vi "DistortImageARGB.vi"(7 "Use Fixed Point Remapping (Default: False)":bool, 8 "error in (no error)":errorcluster, 9 "ARGB Image Destination":refnum<data-value>, 10 "ARGB Image Source":refnum<data-value>, 11 "ImageDistorter":refnum<class "ImageDistorter.lvclass">) -> (0 "error out":errorcluster, 2 "ARGB Image Destination (duplicate)":refnum<data-value>, 3 "ImageDistorter (Duplicate)":refnum<class "ImageDistorter.lvclass">)   [LabVIEW 2020, in "g_ar_toolkit.image.lvlib" / "ImageDistorter.lvclass"]
uses:
  ImageDistorter.lvclass
  ImageDistorter.lvclass/ImageDistorter.ctl
  ccc224f2-fea8-4097-85c8-c2b3fe04188f.vi
  g_ar_toolkit.common/Module Path.vi
  <vilib>/Utility/error.llb/Error Cluster From Error Code.vi
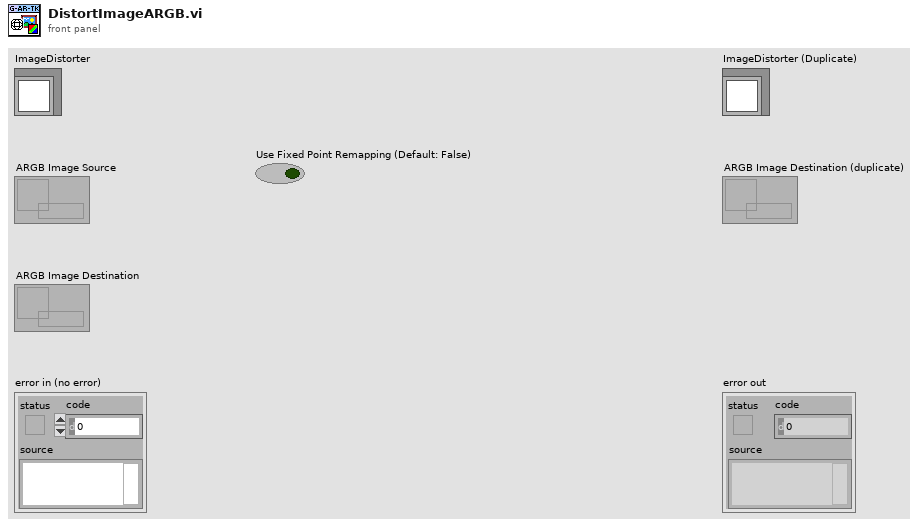
[diagram p1: front panel]
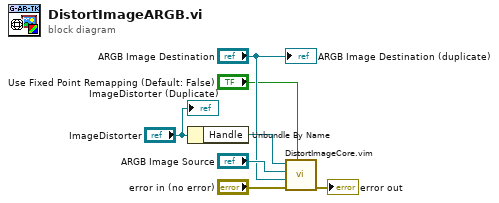
[diagram p0: block diagram]
diagram:
  n1 = Unbundle By Name("ImageDistorter") -> ("Handle"=w6:refnum<data-value>)
  n2 = call "DistortImageCore.vim"("Use Fixed Point remapping"="Use Fixed Point Remapping (Default: False)", "error in (no error)"="error in (no error)", "Destination Image"="ARGB Image Destination", "Source Image"="ARGB Image Source", "Handle"=w6) -> ("error out"=→"error out":errorcluster)  [unwired: 6 in]
  "ImageDistorter (Duplicate)" <- "ImageDistorter"
  "ARGB Image Destination (duplicate)" <- "ARGB Image Destination"
